vi "write_command.vi"(7 "read (T)":bool=TRUE, 8 "error in (no error)":errorcluster, 10 "string to write":string, 11 "LightSourceMH110124MaiTai in":refnum<class "LightSourceMH110124MaiTai.lvclass">) -> (0 "error out":errorcluster, 2 "read string":string, 3 "LightSourceMH110124MaiTai out":refnum<class "LightSourceMH110124MaiTai.lvclass">)   [LabVIEW 2010, in "LightSourceMH110124MaiTai.lvclass"]
uses:
  LightSourceMH110124MaiTai.lvclass
  LightSourceMH110124MaiTai.lvclass/LightSourceMH110124MaiTai.ctl
  common/classes/ErrorController/ErrorController/class_data.vi
  common/classes/ErrorController/ErrorController/ErrorController.lvclass
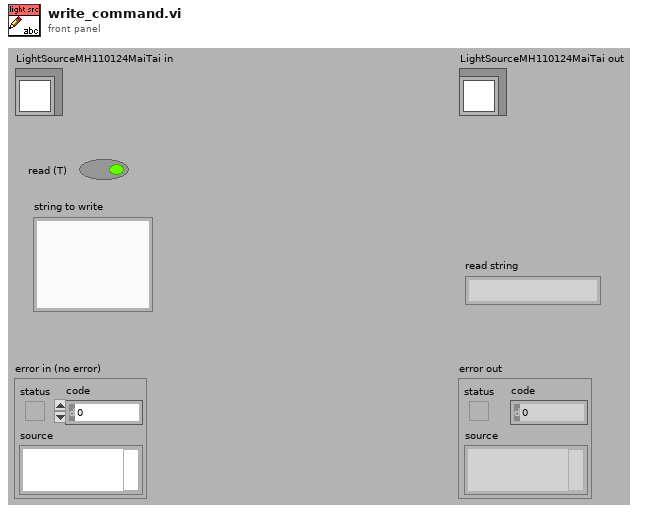
[diagram p1: front panel]
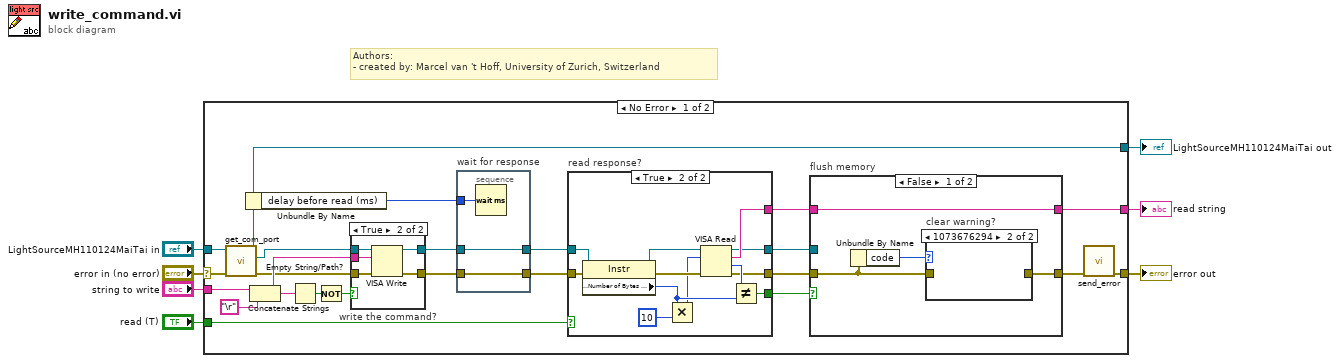
[diagram p0: block diagram]
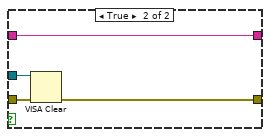
[diagram p3: hidden frame]
diagram:
  # "Authors: \n- created by: Marcel van 't Hoff, University of Zurich, Switzerland"
  n1 = case shown="No Error" "error in (no error)" {
    selector: "error in (no error)" -> [w21 w65]
    tunnel: [w16 w65] -> w6
    tunnel: [w18 w64] -> w4
    tunnel: "LightSourceMH110124MaiTai in" -> [w19 w64]
    tunnel: "string to write" -> [w23 _]
    tunnel: "read (T)" -> [w22 _]
    tunnel: [w9 _] -> w1
    frame No Error {
      n2 = call-dynamic "get_com_port.vi"("error in (no error)"=w21, "LightSourceMH110124MaiTai in"=w19) -> ("error out"=w20:errorcluster, "comm port"=w17:refnum<visa-resource-name>, "LightSourceMH110124MaiTai out"=w18:refnum<class "LightSourceMH110124MaiTai.lvclass">)  [unwired: 7 in]
      n3 = Unbundle By Name(w18) -> ("delay before read (ms)"=w10:u32)
      n4 = Concatenate Strings(w23, "\r") -> (w26:string)
      n5 = Empty String/Path?(string/path=w26) -> (empty?=w25:bool)
      n6 = Not(x=w25) -> (.not. x?=w24:bool)
      n7 = case "write the command?" shown="True" w24 {
        tunnel: [w44 w49] -> w28
        tunnel: w17 -> [w43 w48]
        tunnel: w20 -> [w44 w47]
        tunnel: [w43 w46] -> w30
        tunnel: w26 -> [_ w45]
        frame False {
        }
        frame True {
          n8 = VISA Write(VISA resource name=w48, write buffer=w45, error in (no error)=w47) -> (VISA resource name out=w46:refnum<visa-resource-name>, error out=w49:errorcluster)  [unwired: 1 out]
        }
      }
      n9 = stacked-sequence "wait for response" {
        tunnel: w28 -> [w42]
        tunnel: [w42] -> w29
        tunnel: w30 -> [w41]
        tunnel: [w41] -> w15
        tunnel: w10 -> [w40]
        frame #0 {
          n10 = Wait (ms)(milliseconds to wait=w40) -> ()  [unwired: 1 out]
        }
      }
      n11 = case "read response?" shown="True" w22 {
        tunnel: w29 -> [w51 w61]
        tunnel: [w51 w55] -> w14
        tunnel: w15 -> [w50 w63]
        tunnel: [_ w59] -> w12
        tunnel: [_ w57] -> w11
        tunnel: [w50 w56] -> w13
        frame False {
        }
        frame True {
          n12 = property class="Instr"(reference=w63, error in=w61) -> (reference out=w62:refnum<visa-resource-name>, error out=w60:errorcluster, "Serial Settings:Number of Bytes at Serial Port"=w54:u32)
          n13 = Multiply(x=w54, y=u32 10) -> (x*y=w52:u32)
          n14 = VISA Read(VISA resource name=w62, byte count=w52, error in (no error)=w60) -> (VISA resource name out=w56:refnum<visa-resource-name>, read buffer=w59:string, return count=w58:u32, error out=w55:errorcluster)
          n15 = Not Equal?(x=w58, y=w54) -> (x != y?=w57:bool)
        }
      }
      n16 = case "flush memory" shown="False" w11 {
        tunnel: w14 -> [w32 w39]
        tunnel: w13 -> [_ w38]
        tunnel: [w34 w37] -> w9
        tunnel: w12 -> [w34 w37]
        tunnel: [w31 w36] -> w8
        frame False {
          n17 = Unbundle By Name(w32) -> ("code"=w33:i32)
          n18 = case "clear warning?" shown="1073676294" w33 {
            tunnel: w32 -> [w35 _]
            tunnel: [w35 _] -> w31
            frame Default {
            }
            frame 1073676294 {
            }
          }
        }
        frame True {
          n19 = VISA Clear(VISA resource name=w38, error in (no error)=w39) -> (error out=w36:errorcluster)  [unwired: 1 out]
        }
      }
      n20 = call "send_error.vi"("error in (no error)"=w8) -> ("error out"=w16:errorcluster)  [unwired: 10 in]
    }
    frame Error {
    }
  }
  "error out" <- w6
  "LightSourceMH110124MaiTai out" <- w4
  "read string" <- w1
